vi "Open or Close front panel of caller.vi"(4 "Error Processing":enum16{"Active Errors", "Inactive Errors"}(ring)=enum."Inactive Errors", 5 "Control":enum16{"Open", "Close", "Status", "No Change"}(ring), 6 "error in (no error)":errorcluster, 9 "Is Dialog?":enum16{"Normal", "Dialog Box"}(ring)) -> (0 "error out":errorcluster, 1 "Dialog Box?":bool, 2 "Calling VI":string, 3 "Panel Open?":bool)   [LabVIEW 2013, in "GUI.lvlib"]
doc: "This VI will allow the front panel of the calling VI to be programatically opened or closed, or the status of the panel may be querried. Also this vi may be used to set or revoke the dialog box attribute of the front panel. If not wired, the dialog box attribute defaults to normal window operation (not dialog box)."
uses:
  GUI.lvlib
  Utility/Utility Lib.lvlib
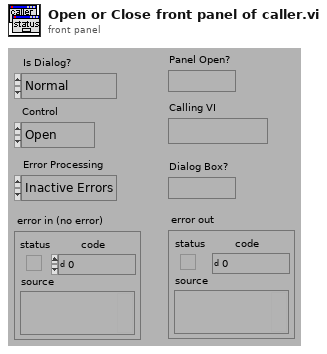
[diagram p1: front panel]
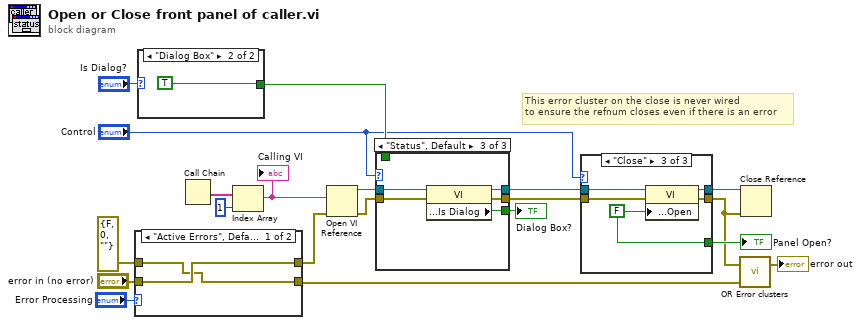
[diagram p0: block diagram]
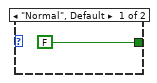
[diagram p2: hidden frame]
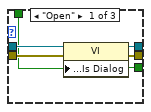
[diagram p3: hidden frame]
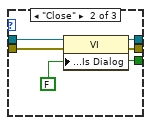
[diagram p4: hidden frame]
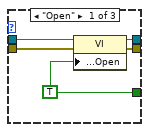
[diagram p6: hidden frame]
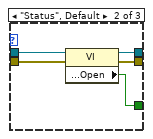
[diagram p7: hidden frame]
diagram:
  # "This error cluster on the close is never wired\nto ensure the refnum closes even if there is an error"
  n1 = case shown="\"Active Errors\", Default" "Error Processing" {
    tunnel: "error in (no error)" -> [w22 w24]
    tunnel: [w22 w23] -> w2
    tunnel: [w21 w24] -> w13
    tunnel: errorcluster {"status"=FALSE, "code"=0, "source"=""} ("error in (no error)") -> [w21 w23]
    frame "Active Errors", Default {
    }
    frame "Inactive Errors" {
    }
  }
  n2 = case shown="\"Dialog Box\"" "Is Dialog?" {
    tunnel: [FALSE TRUE] -> w10
    frame "Normal", Default {
    }
    frame "Dialog Box" {
    }
  }
  n3 = Call Chain() -> (call chain=w20:string[])
  n4 = Index Array(array=w20, index=1) -> (element=w1:string)
  "Calling VI" <- w1
  n5 = Open VI Reference(vi path=w1, error in (no error)=w2) -> (vi reference=w8:refnum<vi>, error out=w7:errorcluster)  [unwired: 1 in, 3 out]
  n6 = case shown="\"Status\", Default" "Control" {
    tunnel: w8 -> [w31 w34 w41]
    tunnel: [w30 w36 w40] -> w6
    tunnel: w7 -> [w29 w33 w38]
    tunnel: [w28 w35 w39] -> w5
    tunnel: [w27 w32 w37] -> w12
    tunnel: w10 -> [w27 _ _]
    frame "Open" {
      n7 = property class="VI"(reference=w31, error in=w29, "Front Panel Window:Is Dialog"=w27) -> (reference out=w30:refnum<vi>, error out=w28:errorcluster)
    }
    frame "Close" {
      w32 = FALSE ("Front Panel Window:Is Dialog")
      n8 = property class="VI"(reference=w34, error in=w33, "Front Panel Window:Is Dialog"=w32) -> (reference out=w36:refnum<vi>, error out=w35:errorcluster)
    }
    frame "Status", Default {
      n9 = property class="VI"(reference=w41, error in=w38) -> (reference out=w40:refnum<vi>, error out=w39:errorcluster, "Front Panel Window:Is Dialog"=w37:bool)
    }
  }
  "Dialog Box?" <- w12
  n10 = case shown="\"Close\"" "Control" {
    tunnel: w6 -> [w45 w47 w52]
    tunnel: [w43 w50 w55] -> w4
    tunnel: w5 -> [w44 w48 w53]
    tunnel: [w46 w51 w56] -> w18
    tunnel: [w42 w49 w54] -> w9
    frame "Open" {
      w46 = TRUE ("Front Panel.Open")
      n11 = property class="VI"(reference=w45, error in=w44, "Front Panel Window:Open"=w46) -> (reference out=w42:refnum<vi>, error out=w43:errorcluster)
    }
    frame "Status", Default {
      n12 = property class="VI"(reference=w47, error in=w48) -> (reference out=w49:refnum<vi>, error out=w50:errorcluster, "Front Panel Window:Open"=w51:bool)
    }
    frame "Close" {
      w56 = FALSE ("Front Panel.Open")
      n13 = property class="VI"(reference=w52, error in=w53, "Front Panel Window:Open"=w56) -> (reference out=w54:refnum<vi>, error out=w55:errorcluster)
    }
  }
  "Panel Open?" <- w18
  n14 = call "OR Error clusters.vi"("error in 2"=w13, "error in 1"=w4) -> ("error out"=→"error out":errorcluster)  [unwired: 1 out]
  n15 = Close Reference(reference=w9, error in (no error)=w4) -> ()  [unwired: 1 out]
